vi "GernateViDoc.vi"() -> ()   [LabVIEW 2020]
panel:
  out "error out":errorcluster
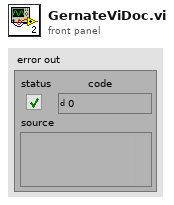
[diagram p1: front panel]
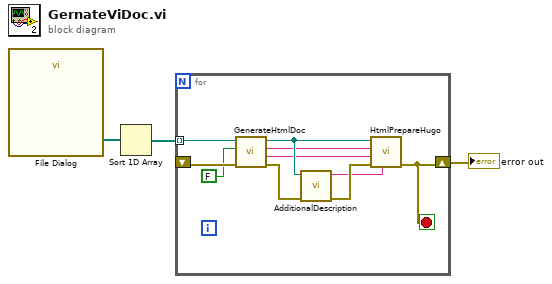
[diagram p0: block diagram]
diagram:
  n1 = call "File Dialog"() -> ("selected paths"=w2:path[])  [unwired: 12 in, 3 out]
  n2 = Sort 1D Array(array=w2) -> (sorted array=w1:path[])
  n3 = for {
    shift-right: [w12] -> w3
    shift-left: _ -> [w13]
    tunnel: w1 -> [w11] mode=indexing
    stop <- w12 stop-if-true
    n4 = call "GenerateHtmlDoc.vi"("error in"=w13, "Clear"=FALSE, "Vi"=w11) -> ("error out"=w9:errorcluster, "Title"=w4:string, "VI Description"=w5:string, "Html Path"=w7:path)  [unwired: 5 in]
    n5 = call "AdditionalDescription.vi"("error in"=w9, "Vi"=w7) -> ("error out"=w8:errorcluster, "Additonal Description"=w6:string)  [unwired: 8 in]
    n6 = call "HtmlPrepareHugo.vi"("Additional Description"=w6, "error in"=w8, "ViTitle"=w4, "ViDescr"=w5, "Html Path"=w7) -> ("error out"=w12:errorcluster)  [unwired: 6 in]
  }
  "error out" <- w3
